vi "PPMS.getMagnet.vi"(8 "error in (no error)":errorcluster, 11 "instrument.PPMS":refnum<class "instrument.PPMS.lvclass">) -> (0 "error out":errorcluster, 2 "Magnet Status":T1, 3 "instrument.PPMS out":refnum<class "instrument.PPMS.lvclass">)   [LabVIEW 2019, in "instrument.PPMS.lvclass"]
uses:
  instrument.PPMS.lvclass
  Typedefs/PPMS.Magnet Status--cluster.ctl
  instrument.PPMS.lvclass/instrument.PPMS.ctl
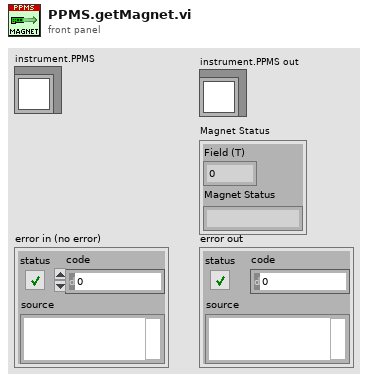
[diagram p1: front panel]
types:
  T1 = typedef "instrument.PPMS.lvclass/PPMS.Magnet Status--cluster.ctl" = cluster{"Field (T)":dbl, "Magnet Status":string}
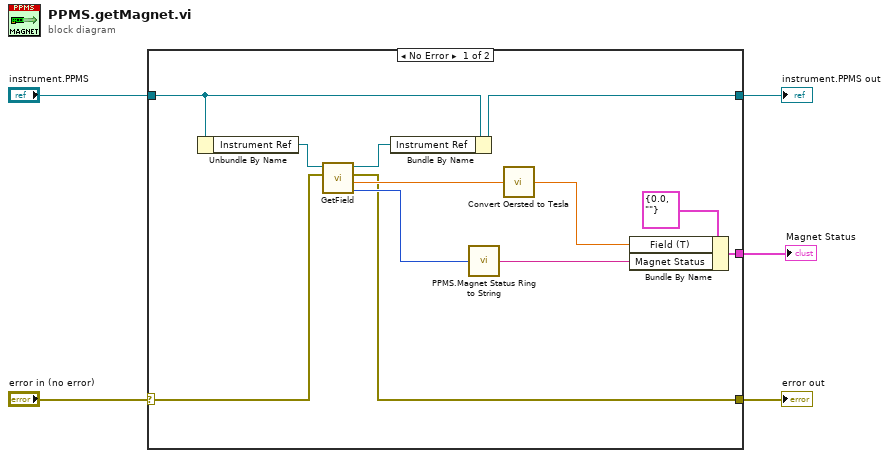
[diagram p0: block diagram]
diagram:
  n1 = case shown="No Error" "error in (no error)" {
    selector: "error in (no error)" -> [w12 w19]
    tunnel: [w7 w19] -> w5
    tunnel: "instrument.PPMS" -> [w14 w18]
    tunnel: [w6 w18] -> w2
    tunnel: [w16 _] -> w1
    frame No Error {
      n2 = Unbundle By Name(w14) -> ("Instrument Ref"=w15:refnum<k24>)
      n3 = call "GetField.vi"("error in (no error)"=w12, "Instrument Ref In"=w15) -> ("Field\nStatus"=w13:i32, "Field"=w11:dbl, "error out"=w7:errorcluster, "Instrument Ref Out"=w8:refnum<k24>)  [unwired: 3 in, 1 out]
      n4 = Bundle By Name(cluster=w14, "Instrument Ref"=w8) -> (w6:refnum<class "instrument.PPMS.lvclass">)
      n5 = call "PPMS.Magnet Status Ring to String.vi"("Field Status"=w13) -> ("Status String"=w9:string)
      n6 = call "Convert Oersted to Tesla.vi"("Field (Oe)"=w11) -> ("Field (T)"=w10:dbl)
      n7 = Bundle By Name(cluster=T1 {"Field (T)"=0.0, "Magnet Status"=""} ("Magnet Status"), "Field (T)"=w10, "Magnet Status"=w9) -> (w16:T1)
    }
    frame Error {
    }
  }
  "Magnet Status" <- w1
  "error out" <- w5
  "instrument.PPMS out" <- w2
